vi "Test TDMS scale.vi"() -> ()   [LabVIEW 2016]
uses:
  <vilib>/Utility/tdmsutil.llb/TDMS Create Scaling Information (Linear).vi
panel:
  in  "y intercect":dbl=-10.0
  in  "scale":dbl=0.1
  in  "Array - Numeric":i16[](array[numeric])=[0, 1, 2]
  in  "File Path Control":path=path "C:/Data/test.tdms"
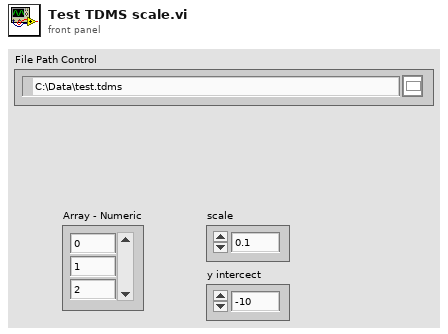
[diagram p1: front panel]
types:
  T1 = enum16{"open", "open or create", "create or replace", "create", "open (read-only)"}
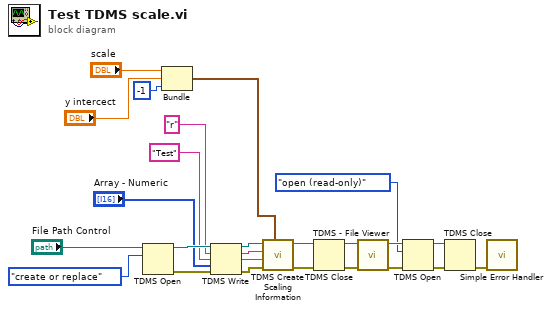
[diagram p0: block diagram]
diagram:
  n1 = TDMS Open(10:T1."create or replace" ("operation (0:open)"), 11:"File Path Control") -> (0:w22:errorcluster, 3:w24:refnum<k34>)  [unwired: 5 in]
  n2 = Bundle("scale"="scale", "y intercect"="y intercect", -1) -> (w7:cluster{"scale":dbl, "y intercect":dbl, i32})  [unwired: 1 in]
  n3 = TDMS Write(0:w24, 5:"r" ("group name"), 7:"Test", 9:"Array - Numeric", 11:w22) -> (4:w6:refnum<k34>, 6:w4:string, 8:w3:string, 15:w2:errorcluster)  [unwired: 1 in]
  n4 = call-poly <vilib>:"TDMS Create Scaling Information.vi"("linear scale"=w7, "error in (no error)"=w2, "channel name"=w3, "group name"=w4, "tdms file"=w6) -> ("error out"=w1:errorcluster, "tdms file out"=w5:refnum<k34>)  [unwired: 2 in, 3 out]
  n5 = TDMS Close(8:w1, 11:w5) -> (0:w21:errorcluster, 3:w20:path)
  n6 = call <vilib>:"TDMS - File Viewer.vi"("error in (no error)"=w21, "file path"=w20) -> ("error out"=w19:errorcluster, "file path out"=w18:path)  [unwired: 4 in]
  n7 = TDMS Open(8:w19, 10:T1."open (read-only)" ("operation (0:open)"), 11:w18) -> (0:w16:errorcluster, 3:w14:refnum<k34>)  [unwired: 4 in]
  n8 = TDMS Close(8:w16, 11:w14) -> (0:w15:errorcluster)  [unwired: 1 out]
  n9 = call <vilib>:"Simple Error Handler.vi"("error in (no error)"=w15) -> ()  [unwired: 4 in, 5 out]
